vi "Write_All_Axis_Home_Data.vi"(6 "Loader Home Data":T1={"Approach Velocity\n(In/Sec)"=1.0, "Creep Velocity\n(In/Sec)"=0.5, "Offset (In)"=0.0625, "OffsetVelocity\n(In/Sec)"=0.5, "AccDec\n(In/Sec/Sec)"=1.0, "Position (In)"=0.0} {"Position (In)" min=0.0 max=1.0 format="%.3f"; "AccDec\n(In/Sec/Sec)" min=0.01 max=20.0 format="%.2f"; "OffsetVelocity\n(In/Sec)" min=0.01 max=2.0 format="%.2f"; "Offset (In)" min=-1.0 max=1.0 format="%.3f"; "Creep Velocity\n(In/Sec)" min=0.5 max=1.0 format="%.2f"; "Approach Velocity\n(In/Sec)" min=0.01 max=2.0 format="%.2f"}, 7 "Z Home Data":T1={"Approach Velocity\n(In/Sec)"=1.0, "Creep Velocity\n(In/Sec)"=0.5, "Offset (In)"=-0.0625, "OffsetVelocity\n(In/Sec)"=0.5, "AccDec\n(In/Sec/Sec)"=1.0, "Position (In)"=5.75} {"Position (In)" format="%.3f"; "AccDec\n(In/Sec/Sec)" min=0.01 max=20.0 format="%.2f"; "OffsetVelocity\n(In/Sec)" min=0.01 max=2.0 format="%.2f"; "Offset (In)" min=-1.0 format="%.3f"; "Creep Velocity\n(In/Sec)" min=0.5 max=1.0 format="%.2f"; "Approach Velocity\n(In/Sec)" min=0.01 max=2.0 format="%.2f"}, 8 "error in (no error)":errorcluster, 9 "Y Home Data":T1={"Approach Velocity\n(In/Sec)"=1.0, "Creep Velocity\n(In/Sec)"=0.5, "Offset (In)"=-0.0625, "OffsetVelocity\n(In/Sec)"=0.5, "AccDec\n(In/Sec/Sec)"=1.0, "Position (In)"=5.9} {"Position (In)" format="%.3f"; "AccDec\n(In/Sec/Sec)" min=0.01 max=20.0 format="%.2f"; "OffsetVelocity\n(In/Sec)" min=0.01 max=2.0 format="%.2f"; "Offset (In)" min=-1.0 max=1.0 format="%.3f"; "Creep Velocity\n(In/Sec)" min=0.5 max=1.0 format="%.2f"; "Approach Velocity\n(In/Sec)" min=0.01 max=2.0 format="%.2f"}, 10 "X Home Data":T2={"Approach Velocity (In/Sec)"=1.0, "Creep Velocity (In/Sec)"=0.5, "Offset (In)"=-0.0625, "OffsetVelocity (In/Sec)"=0.5, "AccDec\n(In/Sec/Sec)"=1.0, "Position (In)"=22.525} {"Position (In)" format="%.3f"; "AccDec\n(In/Sec/Sec)" min=0.01 max=20.0 format="%.2f"; "OffsetVelocity (In/Sec)" min=0.01 max=2.0 format="%.2f"; "Offset (In)" min=-1.0 max=1.0 format="%.3f"; "Creep Velocity (In/Sec)" min=0.5 max=1.0 format="%.2f"; "Approach Velocity (In/Sec)" min=0.01 max=2.0 format="%.2f"}, 11 "TCP Connection Refnum in":refnum<k5>) -> (0 "error out":errorcluster, 3 "TCP Connection Refnum out":refnum<k5>)   [LabVIEW 2010]
uses:
  Motion_Registers Typedef.ctl
  <vilib>/NI Modbus.llb/MB Ethernet Master Query Write Multiple Registers (poly).vi
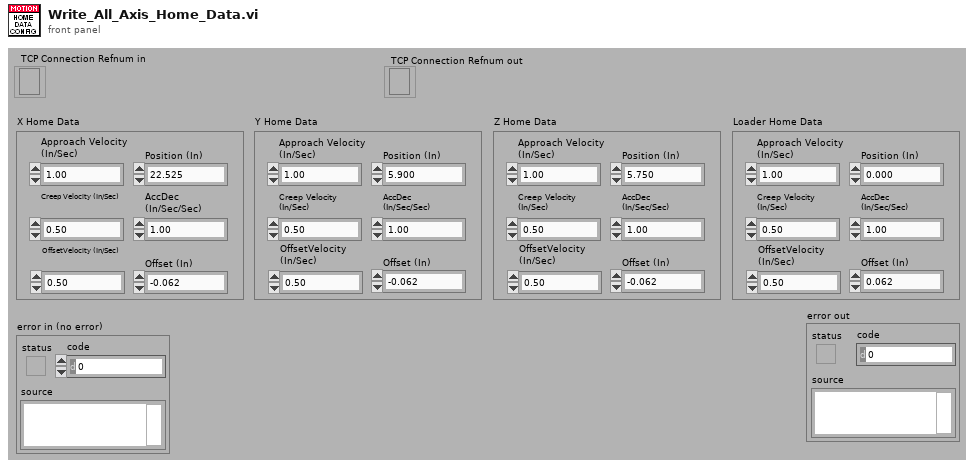
[diagram p1: front panel]
types:
  T1 = cluster{"Approach Velocity\n(In/Sec)":dbl, "Creep Velocity\n(In/Sec)":dbl, "Offset (In)":dbl, "OffsetVelocity\n(In/Sec)":dbl, "AccDec\n(In/Sec/Sec)":dbl, "Position (In)":dbl}
  T2 = cluster{"Approach Velocity (In/Sec)":dbl, "Creep Velocity (In/Sec)":dbl, "Offset (In)":dbl, "OffsetVelocity (In/Sec)":dbl, "AccDec\n(In/Sec/Sec)":dbl, "Position (In)":dbl}
  T3 = typedef "Motion_Registers Typedef.ctl" = u16
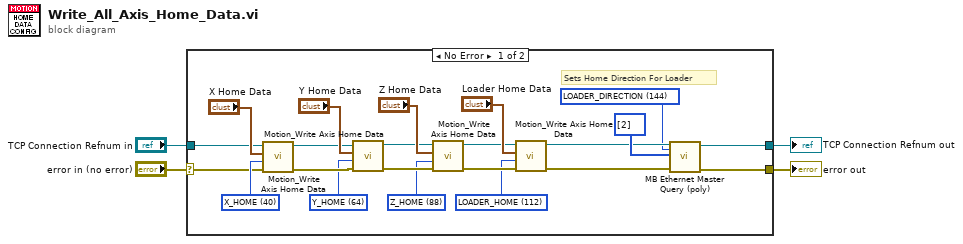
[diagram p0: block diagram]
diagram:
  n1 = case shown="No Error" "error in (no error)" {
    selector: "error in (no error)" -> [w6 w28]
    tunnel: [w8 w27] -> w3
    tunnel: [w7 w28] -> w4
    tunnel: "TCP Connection Refnum in" -> [w5 w27]
    frame No Error {
      w12 = T3 144 items=["GANTRY_MOTION"=20, "X_HOME"=40, "Y_HOME"=64, "Z_HOME"=88, "LOADER_HOME"=112, "LOADER_DIRECTION"=144] ("Registers")
      w11 = T3 112 items=["GANTRY_MOTION"=20, "X_HOME"=40, "Y_HOME"=64, "Z_HOME"=88, "LOADER_HOME"=112, "LOADER_DIRECTION"=144] ("Registers")
      w10 = T3 88 items=["GANTRY_MOTION"=20, "X_HOME"=40, "Y_HOME"=64, "Z_HOME"=88, "LOADER_HOME"=112, "LOADER_DIRECTION"=144] ("Registers")
      w9 = T3 64 items=["GANTRY_MOTION"=20, "X_HOME"=40, "Y_HOME"=64, "Z_HOME"=88, "LOADER_HOME"=112, "LOADER_DIRECTION"=144] ("Registers")
      w13 = T3 40 items=["GANTRY_MOTION"=20, "X_HOME"=40, "Y_HOME"=64, "Z_HOME"=88, "LOADER_HOME"=112, "LOADER_DIRECTION"=144] ("Registers")
      # "Sets Home Direction For Loader"
      n2 = call "Motion_Write Axis Home Data.vi"("error in"=w6, "Register"=w13, "Home Data"="X Home Data", "TCP Connection Refnum in"=w5) -> ("error out"=w17:errorcluster, "TCP Connection Refnum (dup)"=w21:refnum<k5>)  [unwired: 6 in]
      n3 = call "Motion_Write Axis Home Data.vi"("error in"=w17, "Register"=w9, "Home Data"="Y Home Data", "TCP Connection Refnum in"=w21) -> ("error out"=w16:errorcluster, "TCP Connection Refnum (dup)"=w20:refnum<k5>)  [unwired: 6 in]
      n4 = call "Motion_Write Axis Home Data.vi"("error in"=w16, "Register"=w10, "Home Data"="Z Home Data", "TCP Connection Refnum in"=w20) -> ("error out"=w15:errorcluster, "TCP Connection Refnum (dup)"=w19:refnum<k5>)  [unwired: 6 in]
      n5 = call "Motion_Write Axis Home Data.vi"("error in"=w15, "Register"=w11, "Home Data"="Loader Home Data", "TCP Connection Refnum in"=w19) -> ("error out"=w14:errorcluster, "TCP Connection Refnum (dup)"=w18:refnum<k5>)  [unwired: 6 in]
      n6 = call-poly <vilib>:"MB Ethernet Master Query (poly).vi"("TCP Connection Refnum in"=w18, "Starting Address"=w12, "Registers"=u16[] [2], "error in"=w14) -> ("TCP Connection Refnum (dup)"=w8:refnum<k5>, "error out"=w7:errorcluster)  [unwired: 13 in, 1 out]
    }
    frame Error {
    }
  }
  "error out" <- w4
  "TCP Connection Refnum out" <- w3
